vi "系统设置.vi"() -> ()   [LabVIEW 2016]
uses:
  <vilib>/Utility/miscctls.llb/LVPointTypeDef.ctl
  <vilib>/ptbypt/NI_PtbyPt.lvlib
  <vilib>/Utility/config.llb/NI_LVConfig.lvlib
  PLC/PLC.lvlib
panel:
  in  "总磷":bool
  in  "模块启用配置":bool
  in  "短信报警设置":bool
  in  "首页显示设置":bool
  in  "跨度核查":bool
  in  "空白核查":bool
  out "选项卡控件":enum32{"自由设定", "国标协议", "流量设定"}(tab)
  in  "24H周期设置":bool[](xcontrol)
  in  "运行间隔":i16=4 min=1 max=24
  in  "流量阈值":dbl=4.0 min=1.0 max=24.0
  in  "时间阈值":u16=4 min=1 max=24
  in  "周期设置":enum16{"自由设定", "国标协议", "流量设定"}(ring)
  out "x = y?":bool
  in  "质控启动日期":string(combo)="关闭"
  in  "跨度核查时间":u16(ring)=6 items=["00H", "01H", "02H", "03H", "04H", "05H", "06H", "07H", "08H", "09H", "10H", "11H", "12H", "13H", "14H", "15H", "16H", "17H", "18H", "19H", "20H", "21H", "22H", "23H", "关闭"]
  in  "空白核查时间":u16(ring)=2 items=["00H", "01H", "02H", "03H", "04H", "05H", "06H", "07H", "08H", "09H", "10H", "11H", "12H", "13H", "14H", "15H", "16H", "17H", "18H", "19H", "20H", "21H", "22H", "23H", "关闭"]
  in  "CODCr":bool
  in  "总氮":bool
  in  "氨氮":bool
  in  "CODmn":bool
  in  "多参数":bool
  in  "输入密码":dbl
  in  "布尔":bool
  in  "副屏显示设置":bool
  in  "开机启动":bool caption="氨氮禁用"
  in  "运行模式":enum16{"维护模式", "常规模式", "应急模式", "质控模式"}(ring)
  # "注：周期设置分为自由设定和国标协议两种。\n1：选择自由设定情况下：运行间隔将不可选用并变灰色，周期设置可自由手动勾选\n2：选择国标协议情况下：周期时间将由运行间隔选择的时间决定，下方周期设置被禁用并无法手动勾选。\n3：选择流量设定情况下：瞬时流量连续超过流量阈值到达时间阈值设定值，仪器将自动开启测量。"
  # "自动运行启动参数"
  # "质控频次："
  # "零点核查时间："
  # "跨度核查时间："
  # "启动周期设置"
  # "m3/S"
  # "秒"
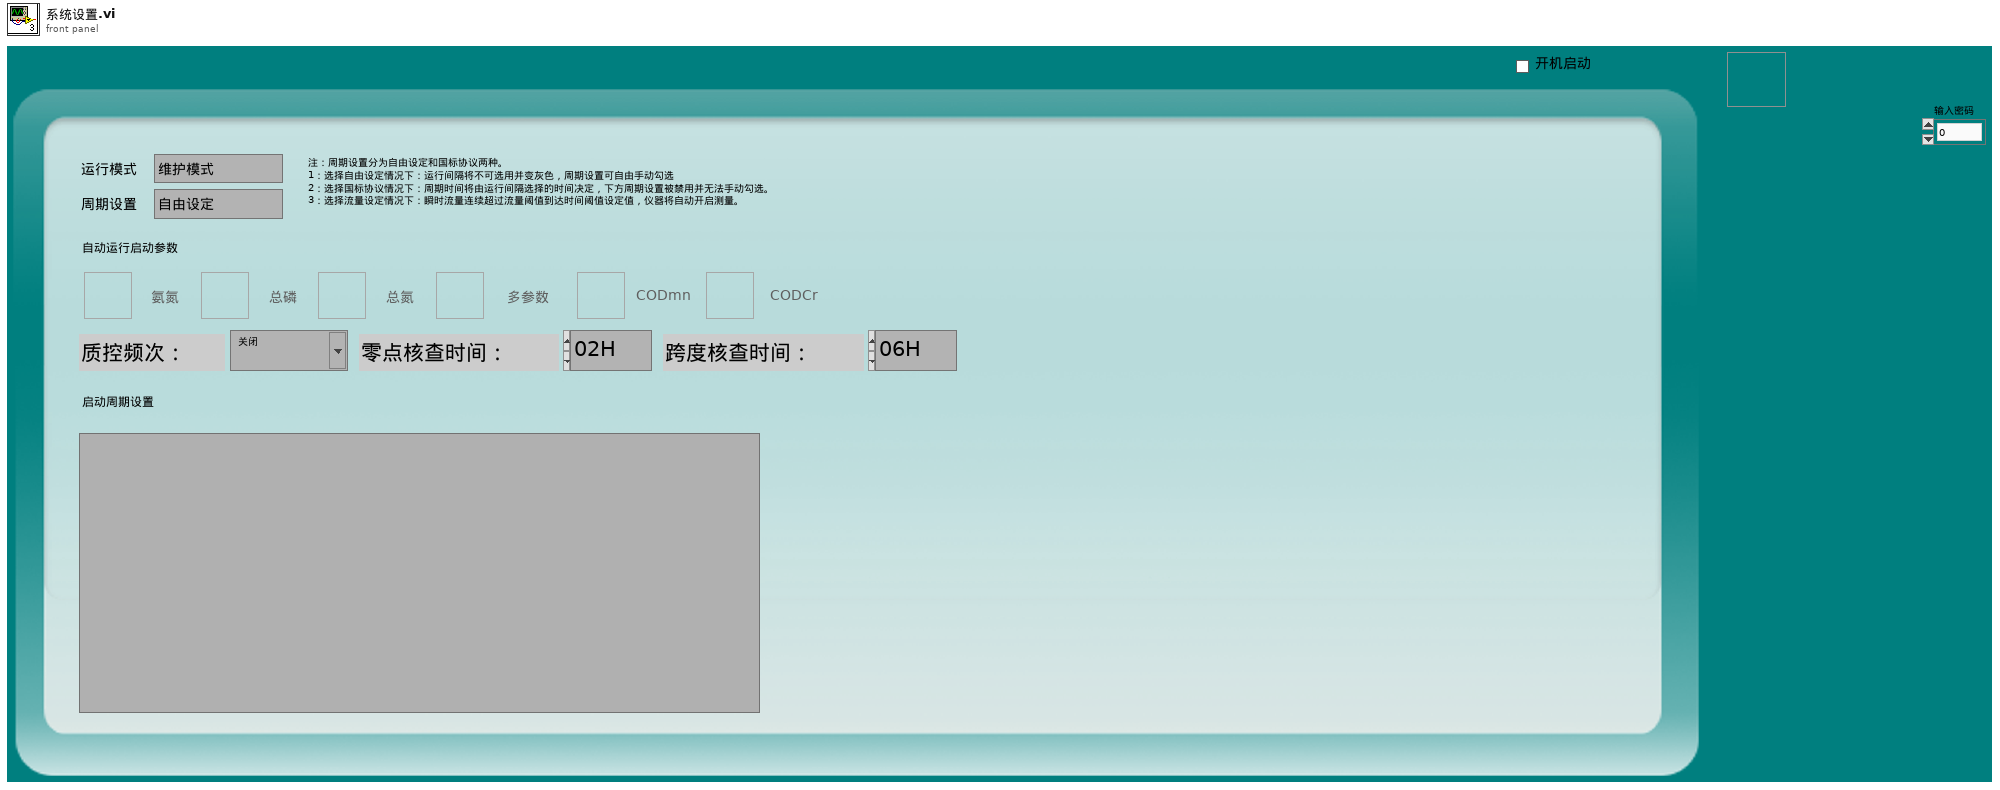
[diagram p1: front panel]
types:
  T1 = typedef "NI_LVConfig.lvlib/Config Data RefNum.ctl" = refnum<k1>
  T2 = typedef "LVPointTypeDef.ctl" = cluster{"Horizontal":i16, "Vertical":i16}
  T3 = enum8{"Enabled", "Disabled", "Disabled and Grayed Out"}
  T4 = enum32{"Bad", "Idle", "Run top level", "Running"}
  T5 = enum32{"Invalid", "Standard", "Closed", "Hidden", "Minimized", "Maximized"}
  T6 = cluster{"运行模式":enum16{"维护模式", "常规模式", "应急模式", "质控模式"}}
  T7 = enum16{"启动测量", "标样核查", "零点核查", "跨度核查", "空白测试", "平行样测试", "加标回收", "空白校准", "标样校准", "初始化（清洗）", "停止测试", "仪器重启", "校时", "模式设置", "测量间隔设置"}
  T8 = cluster{"测量模式":enum16{"水样测量", "标样核查", "零点核查", "跨度核查", "空白测试", "加标回收", "平行样", "校零", "校标"}}
  T9 = cluster{"测试模式":enum16{"正常测试", "集成干预"}, "参数启用":cluster{"氨氮":bool, "总磷":bool, "总氮":bool, "多参数":bool, "CODMn":bool, "CODcr":bool}}
  T10 = cluster{"运行模式":enum16{"维护模式", "常规模式", "应急模式", "质控模式"}, "质控频次":enum16{"关闭", "每天", "星期一", "星期二", "星期三", "星期四", "星期五", "星期六", "星期日"}, "空白核查时间":u16, "跨度核查时间":u16, "24H周期设置":bool[]}
  T11 = typedef "LVDateTimeRec.ctl" = cluster{"秒数的小数部分":dbl, "秒":i32, "分":i32, "时":i32, "日":i32, "月":i32, "年":i32, "天数（周）":i32, "天数（年）":i32, "DST":i32}
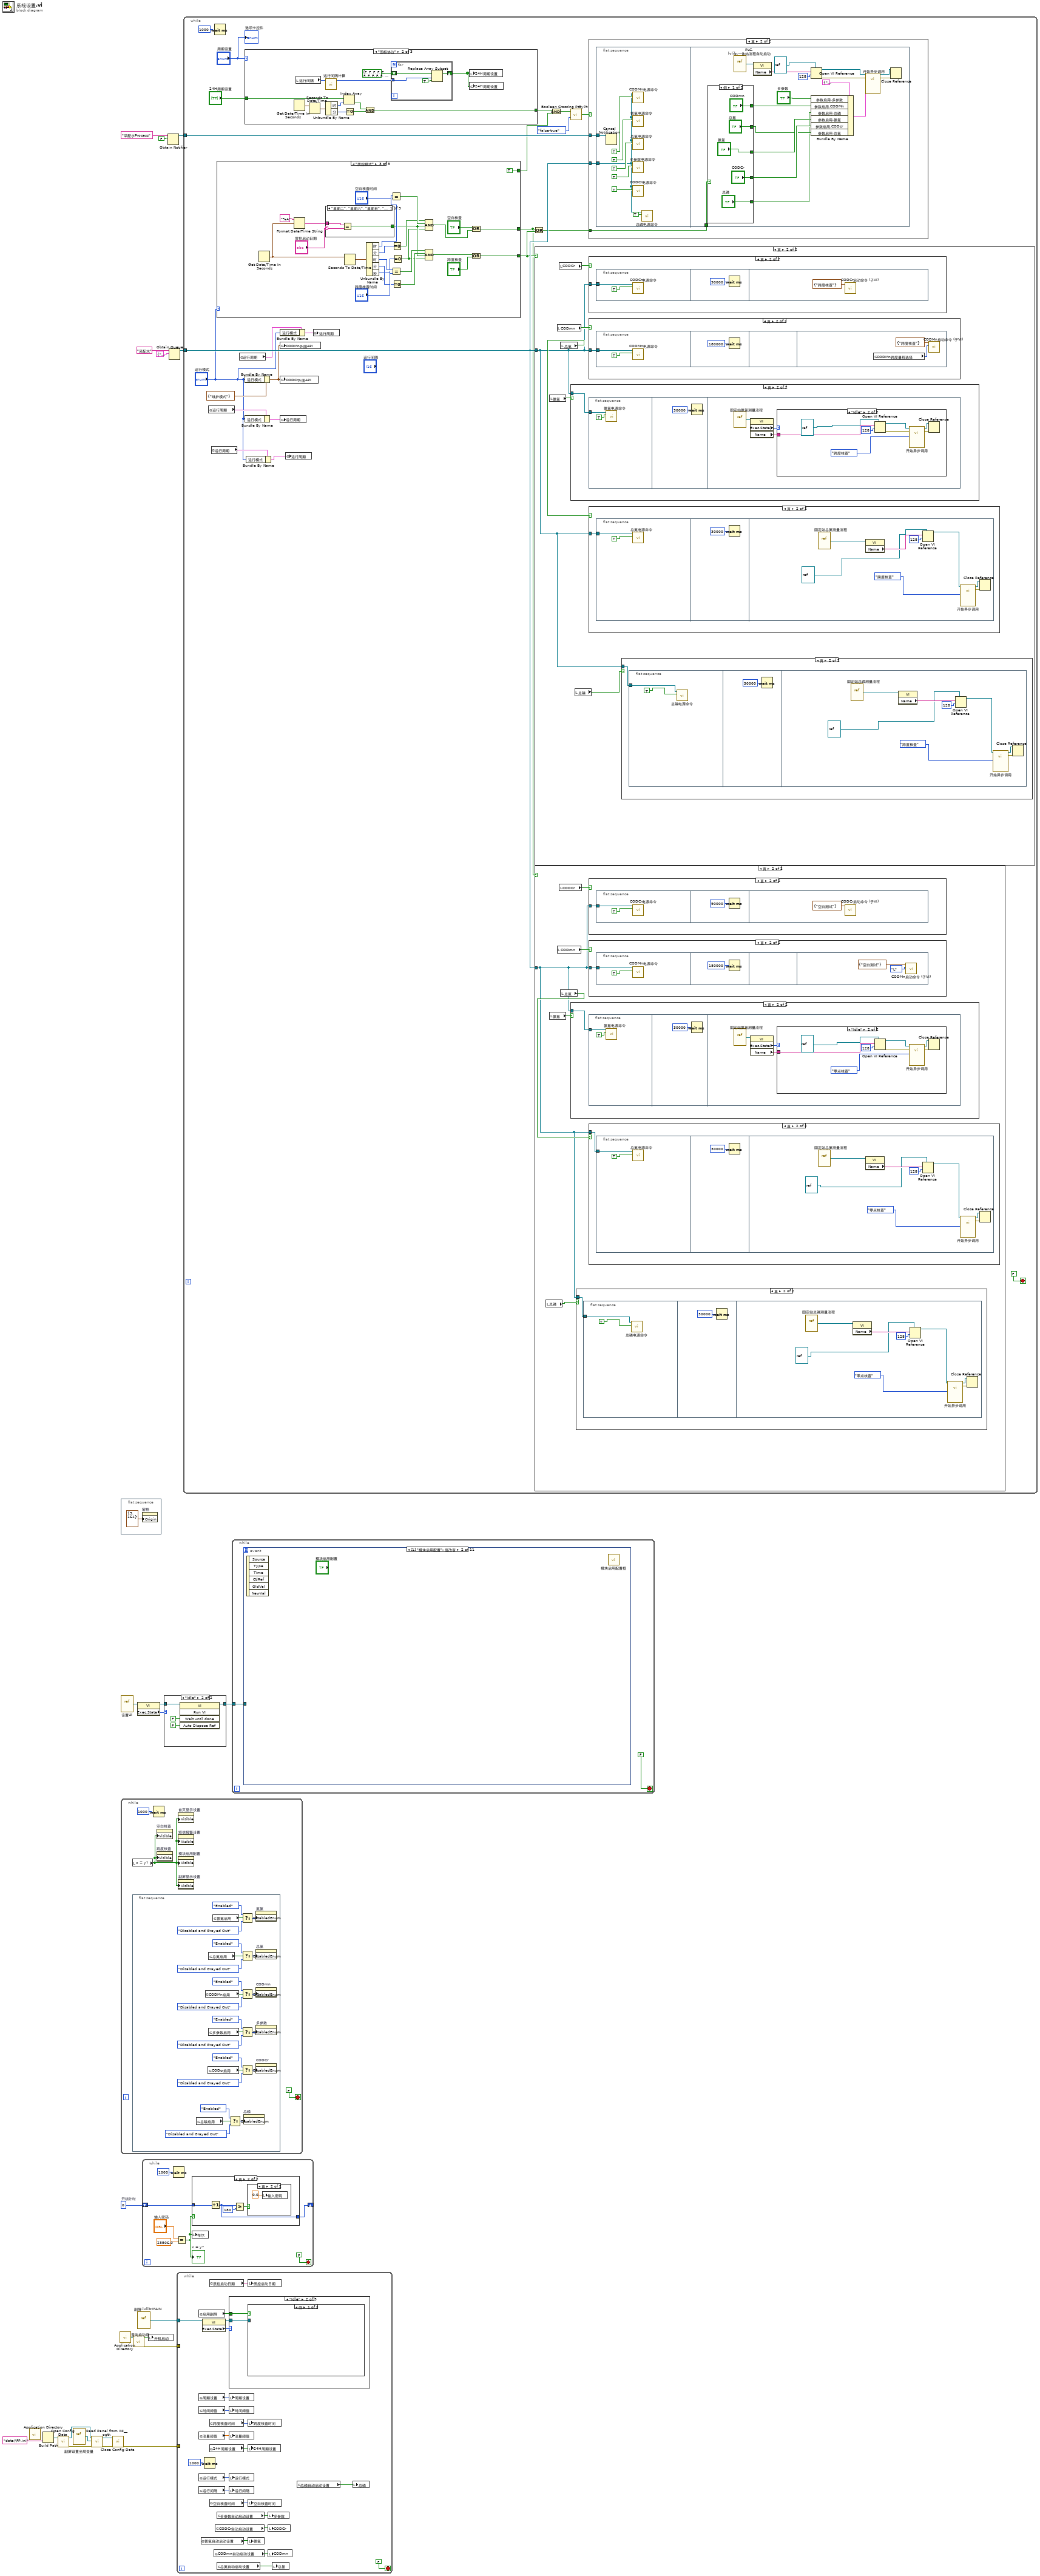
[diagram p0: block diagram]
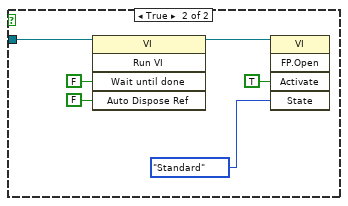
[diagram p6: hidden frame]
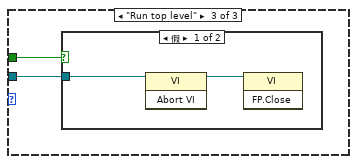
[diagram p7: hidden frame]
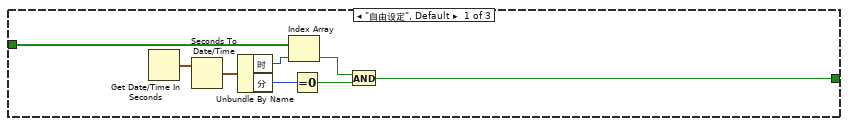
[diagram p9: hidden frame]
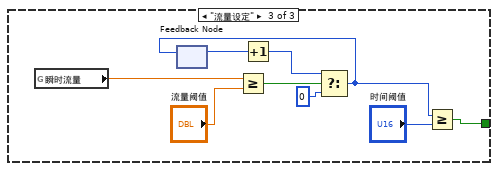
[diagram p10: hidden frame]
diagram:
  w18 = u32 0  # 开锁计时
  n1 = call <vilib>:"Application Directory.vi"() -> ()  [unwired: 1 out]
  n2 = Build Path(name or relative path="data\\FP.ini" ("名称或相对路径")) -> (appended path=w7:path)  [unwired: 1 in]
  n3 = call <vilib>:"Open Config Data.vi"("configuration file path"=w7) -> ("error out"=w6:errorcluster, "refnum"=w3:T1)  [unwired: 8 in, 1 out]
  n4 = vi-ref "副屏设置全局变量.vi"() -> (w4:refnum<vi>)
  n5 = call <userlib>:"Read Panel from INI__ogtk.vi"("error in (no error)"=w6, "VI ref"=w4, "refnum"=w3) -> ("error out"=w5:errorcluster, "refnum out"=w2:T1)  [unwired: 7 in]
  n6 = call <vilib>:"Close Config Data.vi"("error in (no error)"=w5, "refnum"=w2) -> ("error out"=w1:errorcluster)  [unwired: 8 in, 1 out]
  n7 = call <vilib>:"Application Directory.vi"() -> ("Application Directory"=w20:path)
  n8 = flat-sequence {
    frame #0 {
      n9 = property on="窗格" class="Pane"("Origin"=T2 {"Horizontal"=3, "Vertical"=164} ("原点")) -> ()  [unwired: 2 in, 2 out]
    }
  }
  n10 = vi-ref "设置UI.vi"() -> (w13:refnum<vi>)
  n11 = while {
    stop <- FALSE stop-if-true
    n12 = local read "x = y?"() -> (w25:bool)
    n13 = flat-sequence {
      frame #0 {
        n14 = global read "系统设置全局变量.vi" "总磷启用"() -> (w30:bool)
        n15 = global read "系统设置全局变量.vi" "CODMn启用"() -> (w37:bool)
        n16 = global read "系统设置全局变量.vi" "CODcr启用"() -> (w38:bool)
        n17 = global read "系统设置全局变量.vi" "总氮启用"() -> (w39:bool)
        n18 = global read "系统设置全局变量.vi" "多参数启用"() -> (w36:bool)
        n19 = global read "系统设置全局变量.vi" "氨氮启用"() -> (w32:bool)
        n20 = Select(t=T3."Enabled" ("禁用"), s=w30, f=T3."Disabled and Grayed Out" ("禁用")) -> (s? t:f=w31:T3)
        n21 = Select(t=T3."Enabled" ("禁用"), s=w32, f=T3."Disabled and Grayed Out" ("禁用")) -> (s? t:f=w40:T3)
        n22 = Select(t=T3."Enabled" ("禁用"), s=w39, f=T3."Disabled and Grayed Out" ("禁用")) -> (s? t:f=w34:T3)
        n23 = Select(t=T3."Enabled" ("禁用"), s=w37, f=T3."Disabled and Grayed Out" ("禁用")) -> (s? t:f=w41:T3)
        n24 = Select(t=T3."Enabled" ("禁用"), s=w36, f=T3."Disabled and Grayed Out" ("禁用")) -> (s? t:f=w35:T3)
        n25 = Select(t=T3."Enabled" ("禁用"), s=w38, f=T3."Disabled and Grayed Out" ("禁用")) -> (s? t:f=w51:T3)
        n26 = property on="总磷" class="Bool (严格)"("DisabledEnum"=w31) -> ()  [unwired: 2 in, 2 out]
        n27 = property on="氨氮" class="Bool (严格)"("DisabledEnum"=w40) -> ()  [unwired: 2 in, 2 out]
        n28 = property on="总氮" class="Bool (严格)"("DisabledEnum"=w34) -> ()  [unwired: 2 in, 2 out]
        n29 = property on="CODmn" class="Bool (严格)"("DisabledEnum"=w41) -> ()  [unwired: 2 in, 2 out]
        n30 = property on="多参数" class="Bool (严格)"("DisabledEnum"=w35) -> ()  [unwired: 2 in, 2 out]
        n31 = property on="CODCr" class="Bool (严格)"("DisabledEnum"=w51) -> ()  [unwired: 2 in, 2 out]
      }
    }
    n32 = Wait (ms)(milliseconds to wait=u32 1000 ("等待时间（毫秒）")) -> ()  [unwired: 1 out]
    n33 = property on="空白核查" class="Bool"("Visible"=w25) -> ()  [unwired: 2 in, 2 out]
    n34 = property on="跨度核查" class="Bool"("Visible"=w25) -> ()  [unwired: 2 in, 2 out]
    n35 = property on="首页显示设置" class="Bool"("Visible"=w25) -> ()  [unwired: 2 in, 2 out]
    n36 = property on="短信报警设置" class="Bool"("Visible"=w25) -> ()  [unwired: 2 in, 2 out]
    n37 = property on="模块启用配置" class="Bool"("Visible"=w25) -> ()  [unwired: 2 in, 2 out]
    n38 = property on="副屏显示设置" class="Bool"("Visible"=w25) -> ()  [unwired: 2 in, 2 out]
  }
  n39 = call "查询启动项.vi"("启动文件路径"=w20) -> ("error out"=w9:errorcluster, "包含启动项"=w19:bool)  [unwired: 9 in]
  n40 = property class="VI"(reference=w13) -> (reference out=w11:refnum<vi>, "Exec.State"=w12:T4)  [unwired: 1 in, 1 out]
  n41 = vi-ref "副屏.lvlib:MAIN.vi"() -> (w14:refnum<vi>)
  n42 = while {
    shift-right: [w53] -> _
    shift-left: w18 -> [w54]
    stop <- FALSE stop-if-true
    n43 = Wait (ms)(milliseconds to wait=u32 1000 ("等待时间（毫秒）")) -> ()  [unwired: 1 out]
    n44 = Equal?(x="输入密码", y=23506.0) -> (x = y?=w52:bool)
    "x = y?" <- w52
    n45 = case shown="真" w52 {
      tunnel: w54 -> [_ w62]
      tunnel: [_ w61] -> w53
      frame False {
      }
      frame True {
        n46 = Increment(x=w62) -> (x+1=w61:u32)
        n47 = Greater Or Equal?(x=w61, y=u32 180) -> (x >= y?=w59:bool)
        n48 = case shown="真" w59 {
          frame False {
          }
          frame True {
            n49 = local write "输入密码"(0.0 ("输入密码")) -> ()
          }
        }
      }
    }
    n50 = local write "布尔"(w52) -> ()
  }
  n51 = local write "开机启动"(w19) -> ()
  n52 = case shown="\"Idle\"" w12 {
    tunnel: w11 -> [w64 w68]
    tunnel: [w64 w67] -> w10
    frame "Bad", Default {
    }
    frame "Idle" {
      n53 = invoke class="VI" method="Run VI"(reference=w68, "Wait until done"=FALSE ("结束前等待"), "Auto Dispose Ref"=FALSE ("自动销毁引用")) -> (reference out=w67:refnum<vi>)  [unwired: 2 in, 4 out]
    }
  }
  n54 = Obtain Notifier(name (unnamed)="采配水Process" ("名称（未命名）"), notification data type=FALSE) -> (notifier out=w21:refnum<notifier>)  [unwired: 2 in, 2 out]
  n55 = Obtain Queue(name (unnamed)="采配水" ("名称（未命名）"), element data type=cluster{"命令":string, "数据":variant} {"命令"="", "数据"=variant}) -> (queue out=w15:refnum<queue>)  [unwired: 3 in, 2 out]
  n56 = while {
    tunnel: w14 -> [w81]
    tunnel: w9 -> [_]
    tunnel: w1 -> [_]
    stop <- FALSE stop-if-true
    n57 = global read "副屏设置全局变量.vi" "启用副屏"() -> (w79:bool)
    n58 = global read "系统设置全局变量.vi" "周期设置"() -> (w74:enum16{"自由设定", "国标协议", "流量设定"})
    n59 = global read "系统设置全局变量.vi" "时间阈值"() -> (w70:u16)
    n60 = global read "系统设置全局变量.vi" "流量阈值"() -> (w71:dbl)
    n61 = global read "系统设置全局变量.vi" "运行模式"() -> (w72:enum16{"维护模式", "常规模式", "应急模式", "质控模式"})
    n62 = global read "系统设置全局变量.vi" "运行间隔"() -> (w73:i16)
    n63 = global read "系统设置全局变量.vi" "氨氮自动启动设置"() -> (w86:bool)
    n64 = property class="VI"(reference=w81) -> (reference out=w78:refnum<vi>, "Exec.State"=w80:T4)  [unwired: 1 in, 1 out]
    n65 = Wait (ms)(milliseconds to wait=u32 1000 ("等待时间（毫秒）")) -> ()  [unwired: 1 out]
    n66 = global read "系统设置全局变量.vi" "质控启动日期"() -> (w77:string)
    n67 = global read "系统设置全局变量.vi" "跨度核查时间"() -> (w75:u16)
    n68 = global read "系统设置全局变量.vi" "24H周期设置"() -> (w87:bool[])
    n69 = global read "系统设置全局变量.vi" "空白核查时间"() -> (w76:u16)
    n70 = global read "系统设置全局变量.vi" "CODmn自动启动设置"() -> (w83:bool)
    n71 = global read "系统设置全局变量.vi" "CODCr自动启动设置"() -> (w85:bool)
    n72 = global read "系统设置全局变量.vi" "多参数自动启动设置"() -> (w82:bool)
    n73 = global read "系统设置全局变量.vi" "总氮自动启动设置"() -> (w84:bool)
    n74 = case shown="\"Idle\"" w80 {
      tunnel: w79 -> [_ w90 w98]
      tunnel: w78 -> [_ w91 w99]
      frame "Bad", Default {
      }
      frame "Idle" {
        n75 = case shown="假" w90 {
          tunnel: w91 -> [_ w97]
          frame False {
          }
          frame True {
            n76 = invoke class="VI" method="Run VI"(reference=w97, "Wait until done"=FALSE ("结束前等待"), "Auto Dispose Ref"=FALSE ("自动销毁引用")) -> (reference out=w92:refnum<vi>)  [unwired: 2 in, 4 out]
            n77 = invoke class="VI" method="FP.Open"(reference=w92, "Activate"=TRUE ("激活？"), "State"=T5."Standard" ("状态")) -> ()  [unwired: 2 in, 5 out]
          }
        }
      }
      frame "Run top level" {
        n78 = case shown="假" w98 {
          tunnel: w99 -> [w100 _]
          frame False {
            n79 = invoke class="VI" method="Abort VI"(reference=w100) -> (reference out=w101:refnum<vi>)  [unwired: 2 in, 2 out]
            n80 = invoke class="VI" method="FP.Close"(reference=w101) -> ()  [unwired: 2 in, 3 out]
          }
          frame True {
          }
        }
      }
    }
    n81 = local write "周期设置"(w74) -> ()
    n82 = local write "时间阈值"(w70) -> ()
    n83 = local write "流量阈值"(w71) -> ()
    n84 = local write "运行模式"(w72) -> ()
    n85 = local write "运行间隔"(w73) -> ()
    n86 = local write "质控启动日期"(w77) -> ()
    n87 = local write "跨度核查时间"(w75) -> ()
    n88 = local write "24H周期设置"(w87) -> ()
    n89 = local write "空白核查时间"(w76) -> ()
    n90 = local write "氨氮"(w86) -> ()
    n91 = local write "多参数"(w82) -> ()
    n92 = local write "CODCr"(w85) -> ()
    n93 = local write "CODmn"(w83) -> ()
    n94 = local write "总氮"(w84) -> ()
    n95 = global read "系统设置全局变量.vi" "总磷自动启动设置"() -> (w69:bool)
    n96 = local write "总磷"(w69) -> ()
  }
  n97 = while {
    tunnel: w21 -> [w122]
    tunnel: w15 -> [w118]
    stop <- FALSE stop-if-true
    n98 = global read "总氮断电保存全局变量.vi" "运行周期"() -> (w106:T10)
    n99 = global read "总磷断电保存全局变量.vi" "运行周期"() -> (w104:T10)
    n100 = Wait (ms)(milliseconds to wait=u32 1000 ("等待时间（毫秒）")) -> ()  [unwired: 1 out]
    n101 = case shown="\"质控模式\"" "运行模式" {
      tunnel: [_ _ w304] -> w111
      tunnel: [_ _ w308] -> w110
      tunnel: [_ TRUE TRUE] -> w115
      frame "维护模式", Default {
      }
      frame "常规模式" {
      }
      frame "质控模式" {
        n102 = Get Date/Time In Seconds() -> (seconds since 1Jan1904=w315:timestamp)
        n103 = Format Date/Time String(time format string (%c)="%A" ("时间格式字符串(%c)"), seconds (now)=w315) -> (date/time string=w313:string)  [unwired: 1 in]
        n104 = case shown="\"星期二\", \"星期六\", \"星期日\", \"星期三\", \"星期四\", \"星期五\", \"星期一\"" "质控启动日期" {
          selector: "质控启动日期" -> [w331 _ _]
          tunnel: [w330 TRUE FALSE] -> w316
          tunnel: w313 -> [w329 _ _]
          frame "星期二", "星期六", "星期日", "星期三", "星期四", "星期五", "星期一" {
            n105 = Equal?(x=w329, y=w331) -> (x = y?=w330:bool)
          }
          frame "每天" {
          }
          frame "关闭", Default {
          }
        }
        n106 = Seconds To Date/Time(time stamp (now)=w315) -> (date time rec=w328:T11)  [unwired: 1 in]
        n107 = Unbundle By Name(w328) -> ("时"=w327:i32, "分"=w325:i32, "时"=w321:i32, "分"=w320:i32, "秒"=w312:i32)
        n108 = Equal?(x=w327, y="空白核查时间") -> (x = y?=w324:bool)
        n109 = Equal?(x=w321, y="跨度核查时间") -> (x = y?=w319:bool)
        n110 = Equal To 0?(x=w325) -> (x = 0?=w323:bool)
        n111 = Equal To 0?(x=w320) -> (x = 0?=w318:bool)
        n112 = Equal To 0?(x=w312) -> (x = 0?=w311:bool)
        n113 = Compound Arithmetic op=AND ("复合运算")(w323, w324, w316, w311) -> (w309:bool)
        n114 = Compound Arithmetic op=AND ("复合运算")(w319, w318, w316, w311) -> (w306:bool)
        n115 = Or(x="空白核查", y=w309) -> (x .or. y?=w308:bool)
        n116 = Or(x=w306, y="跨度核查") -> (x .or. y?=w304:bool)
      }
    }
    n117 = global read "氨氮断电保存全局变量.vi" "运行周期"() -> (w108:T10)
    n118 = case shown="\"国标协议\"" "周期设置" {
      tunnel: [w126 w133 w149] -> w114
      tunnel: "24H周期设置" -> [w125 w134 _]
      frame "自由设定", Default {
        n119 = Get Date/Time In Seconds() -> (seconds since 1Jan1904=w127:timestamp)
        n120 = Seconds To Date/Time(time stamp (now)=w127) -> (date time rec=w128:T11)  [unwired: 1 in]
        n121 = Unbundle By Name(w128) -> ("时"=w131:i32, "分"=w129:i32)
        n122 = Index Array(array=w125, index=w131) -> (element=w132:bool)
        n123 = Equal To 0?(x=w129) -> (x = 0?=w130:bool)
        n124 = And(x=w132, y=w130) -> (x .and. y?=w126:bool)
      }
      frame "国标协议" {
        n125 = Get Date/Time In Seconds() -> (seconds since 1Jan1904=w135:timestamp)
        n126 = local read "运行间隔"() -> (w144:i16)
        n127 = Seconds To Date/Time(time stamp (now)=w135) -> (date time rec=w136:T11)  [unwired: 1 in]
        n128 = call "运行间隔计算.vi"("运行周期"=w144) -> ("数组"=w143:i32[])  [unwired: 10 in]
        n129 = Unbundle By Name(w136) -> ("时"=w139:i32, "分"=w137:i32)
        n130 = Index Array(array=w134, index=w139) -> (element=w140:bool)
        n131 = Equal To 0?(x=w137) -> (x = 0?=w138:bool)
        n132 = And(x=w140, y=w138) -> (x .and. y?=w133:bool)
        n133 = for {
          tunnel: w143 -> [w147] mode=indexing
          shift-right: [w145] -> w141
          shift-left: bool[] [FALSE, FALSE, FALSE, FALSE, FALSE, FALSE, FALSE, FALSE, FALSE, FALSE, FALSE, FALSE, FALSE, FALSE, FALSE, FALSE, FALSE, FALSE, FALSE, FALSE, FALSE, FALSE, FALSE, FALSE] ("24H周期设置") -> [w148]
          n134 = Replace Array Subset(array=w148, new element=TRUE ("新元素/子数组"), index=w147) -> (w145:bool[])
        }
        n135 = local write "24H周期设置"(w141) -> ()
        n136 = global write "系统设置全局变量.vi" "24H周期设置"(w141) -> ()
      }
      frame "流量设定" {
        n137 = global read "流量计全局变量.vi" "瞬时流量"() -> (w157:dbl)
        n138 = feedback #1() -> (w154:i16)  [unwired: 1 in]
        n139 = Greater Or Equal?(x=w157, y="流量阈值") -> (x >= y?=w152:bool)
        n140 = Increment(x=w154) -> (x+1=w153:i16)
        n141 = Select(t=w153, s=w152, f=i16 0) -> (s? t:f=w151:i16)
        n142 = feedback-in #1(w151) -> ()
        n143 = Greater Or Equal?(x=w151, y="时间阈值") -> (x >= y?=w149:bool)
      }
    }
    n144 = Bundle By Name(cluster=T6 {"运行模式"=enum."维护模式"} ("外围API"), "运行模式"="运行模式") -> (w112:T6)
    n145 = Bundle By Name(cluster=w106, "运行模式"="运行模式") -> (w105:T10)
    n146 = Bundle By Name(cluster=w104, "运行模式"="运行模式") -> (w103:T10)
    n147 = Bundle By Name(cluster=w108, "运行模式"="运行模式") -> (w107:T10)
    n148 = global write "CODMN外部API.vi" "CODMn外围API"(w112) -> ()
    n149 = global write "CODCr外部API.vi" "CODCr外围API"(w112) -> ()
    n150 = global write "总氮断电保存全局变量.vi" "运行周期"(w105) -> ()
    n151 = global write "总磷断电保存全局变量.vi" "运行周期"(w103) -> ()
    n152 = global write "氨氮断电保存全局变量.vi" "运行周期"(w107) -> ()
    n153 = Or(x=w110, y=w111) -> (x .or. y?=w109:bool)
    n154 = case shown="真" w111 {
      tunnel: w118 -> [_ w159]
      frame False {
      }
      frame True {
        n155 = local read "氨氮"() -> (w163:bool)
        n156 = local read "CODmn"() -> (w161:bool)
        n157 = local read "CODCr"() -> (w160:bool)
        n158 = local read "总氮"() -> (w162:bool)
        n159 = case shown="真" w163 {
          tunnel: w159 -> [_ w199]
          frame False {
          }
          frame True {
            n160 = flat-sequence {
              tunnel: w199 -> [w200]
              frame #0 {
                n161 = call "氨氮电源命令.vi"("通电/断电"=TRUE, "队列"=w200) -> ()  [unwired: 9 in, 1 out]
              }
              frame #1 {
                n162 = Wait (ms)(milliseconds to wait=u32 30000 ("等待时间（毫秒）")) -> ()  [unwired: 1 out]
              }
              frame #2 {
                n163 = vi-ref "固定站氨氮测量流程.vi"() -> (w205:refnum<vi>)
                n164 = property class="VI"(reference=w205) -> ("Exec.State"=w203:T4, "Name"=w204:string)  [unwired: 1 in, 2 out]
                n165 = case shown="\"Idle\"" w203 {
                  tunnel: w204 -> [_ w210]
                  frame "Bad", Default {
                  }
                  frame "Idle" {
                    n166 = Open VI Reference(type specifier VI Refnum (for type only)=refnum<vi> refnum, vi path=w210, options=128 ("选项")) -> (vi reference=w208:refnum<vi>, error out=w211:errorcluster)  [unwired: 3 in]
                    n167 = call-by-ref "开始异步调用"(reference=w208, error in=w211, "控制命令"=T7."跨度核查") -> (reference out=w212:refnum<vi>, error out=w213:errorcluster)  [unwired: 11 in]
                    n168 = Close Reference(reference=w212, error in (no error)=w213) -> ()  [unwired: 1 out]
                  }
                }
              }
            }
          }
        }
        n169 = local read "总磷"() -> (w158:bool)
        n170 = case shown="真" w160 {
          tunnel: w159 -> [_ w176]
          frame False {
          }
          frame True {
            n171 = flat-sequence {
              tunnel: w176 -> [w177]
              frame #0 {
                n172 = call "CODCr电源命令.vi"("通电/断电"=TRUE, "队列"=w177) -> ()  [unwired: 9 in, 1 out]
              }
              frame #1 {
                n173 = Wait (ms)(milliseconds to wait=u32 90000 ("等待时间（毫秒）")) -> ()  [unwired: 1 out]
              }
              frame #2 {
                n174 = call "CODCr启动命令 (子VI).vi"("启动测量模式"=T8 {"测量模式"=enum."跨度核查"}) -> ()  [unwired: 11 in]
              }
            }
          }
        }
        n175 = case shown="真" w161 {
          tunnel: w159 -> [_ w181]
          frame False {
          }
          frame True {
            n176 = flat-sequence {
              tunnel: w181 -> [w182]
              frame #0 {
                n177 = call "CODMn电源命令.vi"("通电/断电"=TRUE, "队列"=w182) -> ()  [unwired: 9 in, 1 out]
              }
              frame #1 {
                n178 = Wait (ms)(milliseconds to wait=u32 180000 ("等待时间（毫秒）")) -> ()  [unwired: 1 out]
              }
              frame #2 {
              }
              frame #3 {
                n179 = global read "CODMn断电保存全局变量.vi" "CODMn跨度量程选择"() -> (w185:enum32{"H", "L", "AUTO"})
                n180 = call "CODMn启动命令 (子VI).vi"("CODMn量程切换"=w185, "启动测量模式"=T8 {"测量模式"=enum."跨度核查"}) -> ()  [unwired: 10 in]
              }
            }
          }
        }
        n181 = case shown="真" w162 {
          tunnel: w159 -> [_ w187]
          frame False {
          }
          frame True {
            n182 = flat-sequence {
              tunnel: w187 -> [w189]
              frame #0 {
                n183 = call "总氮电源命令.vi"("通电/断电"=TRUE, "队列"=w189) -> ()  [unwired: 9 in, 1 out]
              }
              frame #1 {
                n184 = Wait (ms)(milliseconds to wait=u32 30000 ("等待时间（毫秒）")) -> ()  [unwired: 1 out]
              }
              frame #2 {
                n185 = vi-ref "固定站总氮测量流程.vi"() -> (w196:refnum<vi>)
                n186 = property class="VI"(reference=w196) -> ("Name"=w197:string)  [unwired: 1 in, 2 out]
                n187 = Open VI Reference(type specifier VI Refnum (for type only)=refnum<vi> refnum, vi path=w197, options=128 ("选项")) -> (vi reference=w195:refnum<vi>)  [unwired: 3 in, 1 out]
                n188 = call-by-ref "开始异步调用"(reference=w195, "控制命令"=T7."跨度核查") -> (reference out=w194:refnum<vi>, error out=w193:errorcluster)  [unwired: 12 in]
                n189 = Close Reference(reference=w194, error in (no error)=w193) -> ()  [unwired: 1 out]
              }
            }
          }
        }
        n190 = case shown="真" w158 {
          tunnel: w159 -> [_ w164]
          frame False {
          }
          frame True {
            n191 = flat-sequence {
              tunnel: w164 -> [w166]
              frame #0 {
                n192 = call "总磷电源命令.vi"("通电/断电"=TRUE, "队列"=w166) -> ()  [unwired: 9 in, 1 out]
              }
              frame #1 {
                n193 = Wait (ms)(milliseconds to wait=u32 30000 ("等待时间（毫秒）")) -> ()  [unwired: 1 out]
              }
              frame #2 {
                n194 = vi-ref "固定站总磷测量流程.vi"() -> (w173:refnum<vi>)
                n195 = property class="VI"(reference=w173) -> ("Name"=w174:string)  [unwired: 1 in, 2 out]
                n196 = Open VI Reference(type specifier VI Refnum (for type only)=refnum<vi> refnum, vi path=w174, options=128 ("选项")) -> (vi reference=w172:refnum<vi>)  [unwired: 3 in, 1 out]
                n197 = call-by-ref "开始异步调用"(reference=w172, "控制命令"=T7."跨度核查") -> (reference out=w171:refnum<vi>, error out=w170:errorcluster)  [unwired: 12 in]
                n198 = Close Reference(reference=w171, error in (no error)=w170) -> ()  [unwired: 1 out]
              }
            }
          }
        }
      }
    }
    n199 = case shown="真" w110 {
      tunnel: w118 -> [_ w215]
      frame False {
      }
      frame True {
        n200 = local read "总磷"() -> (w214:bool)
        n201 = local read "氨氮"() -> (w219:bool)
        n202 = local read "CODmn"() -> (w217:bool)
        n203 = local read "CODCr"() -> (w216:bool)
        n204 = local read "总氮"() -> (w218:bool)
        n205 = case shown="真" w219 {
          tunnel: w215 -> [_ w255]
          frame False {
          }
          frame True {
            n206 = flat-sequence {
              tunnel: w255 -> [w256]
              frame #0 {
                n207 = call "氨氮电源命令.vi"("通电/断电"=TRUE, "队列"=w256) -> ()  [unwired: 9 in, 1 out]
              }
              frame #1 {
                n208 = Wait (ms)(milliseconds to wait=u32 30000 ("等待时间（毫秒）")) -> ()  [unwired: 1 out]
              }
              frame #2 {
                n209 = vi-ref "固定站氨氮测量流程.vi"() -> (w261:refnum<vi>)
                n210 = property class="VI"(reference=w261) -> ("Exec.State"=w259:T4, "Name"=w260:string)  [unwired: 1 in, 2 out]
                n211 = case shown="\"Idle\"" w259 {
                  tunnel: w260 -> [_ w266]
                  frame "Bad", Default {
                  }
                  frame "Idle" {
                    n212 = Open VI Reference(type specifier VI Refnum (for type only)=refnum<vi> refnum, vi path=w266, options=128 ("选项")) -> (vi reference=w264:refnum<vi>, error out=w267:errorcluster)  [unwired: 3 in]
                    n213 = call-by-ref "开始异步调用"(reference=w264, error in=w267, "控制命令"=T7."零点核查") -> (reference out=w268:refnum<vi>, error out=w269:errorcluster)  [unwired: 11 in]
                    n214 = Close Reference(reference=w268, error in (no error)=w269) -> ()  [unwired: 1 out]
                  }
                }
              }
            }
          }
        }
        n215 = case shown="真" w214 {
          tunnel: w215 -> [_ w220]
          frame False {
          }
          frame True {
            n216 = flat-sequence {
              tunnel: w220 -> [w222]
              frame #0 {
                n217 = call "总磷电源命令.vi"("通电/断电"=TRUE, "队列"=w222) -> ()  [unwired: 9 in, 1 out]
              }
              frame #1 {
                n218 = Wait (ms)(milliseconds to wait=u32 30000 ("等待时间（毫秒）")) -> ()  [unwired: 1 out]
              }
              frame #2 {
                n219 = vi-ref "固定站总磷测量流程.vi"() -> (w229:refnum<vi>)
                n220 = property class="VI"(reference=w229) -> ("Name"=w230:string)  [unwired: 1 in, 2 out]
                n221 = Open VI Reference(type specifier VI Refnum (for type only)=refnum<vi> refnum, vi path=w230, options=128 ("选项")) -> (vi reference=w228:refnum<vi>)  [unwired: 3 in, 1 out]
                n222 = call-by-ref "开始异步调用"(reference=w228, "控制命令"=T7."零点核查") -> (reference out=w227:refnum<vi>, error out=w226:errorcluster)  [unwired: 12 in]
                n223 = Close Reference(reference=w227, error in (no error)=w226) -> ()  [unwired: 1 out]
              }
            }
          }
        }
        n224 = case shown="真" w216 {
          tunnel: w215 -> [_ w232]
          frame False {
          }
          frame True {
            n225 = flat-sequence {
              tunnel: w232 -> [w233]
              frame #0 {
                n226 = call "CODCr电源命令.vi"("通电/断电"=TRUE, "队列"=w233) -> ()  [unwired: 9 in, 1 out]
              }
              frame #1 {
                n227 = Wait (ms)(milliseconds to wait=u32 90000 ("等待时间（毫秒）")) -> ()  [unwired: 1 out]
              }
              frame #2 {
                n228 = call "CODCr启动命令 (子VI).vi"("启动测量模式"=T8 {"测量模式"=enum."空白测试"}) -> ()  [unwired: 11 in]
              }
            }
          }
        }
        n229 = case shown="真" w217 {
          tunnel: w215 -> [_ w237]
          frame False {
          }
          frame True {
            n230 = flat-sequence {
              tunnel: w237 -> [w238]
              frame #0 {
                n231 = call "CODMn电源命令.vi"("通电/断电"=TRUE, "队列"=w238) -> ()  [unwired: 9 in, 1 out]
              }
              frame #1 {
                n232 = Wait (ms)(milliseconds to wait=u32 180000 ("等待时间（毫秒）")) -> ()  [unwired: 1 out]
              }
              frame #2 {
              }
              frame #3 {
                n233 = call "CODMn启动命令 (子VI).vi"("CODMn量程切换"=enum32{"H", "L", "AUTO"}."L", "启动测量模式"=T8 {"测量模式"=enum."空白测试"}) -> ()  [unwired: 10 in]
              }
            }
          }
        }
        n234 = case shown="真" w218 {
          tunnel: w215 -> [_ w243]
          frame False {
          }
          frame True {
            n235 = flat-sequence {
              tunnel: w243 -> [w245]
              frame #0 {
                n236 = call "总氮电源命令.vi"("通电/断电"=TRUE, "队列"=w245) -> ()  [unwired: 9 in, 1 out]
              }
              frame #1 {
                n237 = Wait (ms)(milliseconds to wait=u32 30000 ("等待时间（毫秒）")) -> ()  [unwired: 1 out]
              }
              frame #2 {
                n238 = vi-ref "固定站总氮测量流程.vi"() -> (w252:refnum<vi>)
                n239 = property class="VI"(reference=w252) -> ("Name"=w253:string)  [unwired: 1 in, 2 out]
                n240 = Open VI Reference(type specifier VI Refnum (for type only)=refnum<vi> refnum, vi path=w253, options=128 ("选项")) -> (vi reference=w251:refnum<vi>)  [unwired: 3 in, 1 out]
                n241 = call-by-ref "开始异步调用"(reference=w251, "控制命令"=T7."零点核查") -> (reference out=w250:refnum<vi>, error out=w249:errorcluster)  [unwired: 12 in]
                n242 = Close Reference(reference=w250, error in (no error)=w249) -> ()  [unwired: 1 out]
              }
            }
          }
        }
      }
    }
    n243 = And(x=w114, y=w115) -> (x .and. y?=w113:bool)
    n244 = call <vilib>:"Boolean Crossing PtByPt.vi"("direction"=enum16{"either", "false-true", "true-false"}."false-true", "input"=w113) -> ("crossing"=w120:bool)  [unwired: 1 in]
    n245 = case shown="真" w120 {
      tunnel: w122 -> [_ w272]
      tunnel: w118 -> [_ w271]
      tunnel: w109 -> [_ w270]
      frame False {
      }
      frame True {
        n246 = flat-sequence {
          tunnel: w272 -> [w280]
          tunnel: w271 -> [w274]
          tunnel: w270 -> [w286]
          frame #0 {
            n247 = Cancel Notification(0:w280) -> ()  [unwired: 1 in, 3 out]
            n248 = call "CODMn电源命令.vi"("通电/断电"=TRUE, "队列"=w274) -> ()  [unwired: 9 in, 1 out]
            n249 = call "氨氮电源命令.vi"("通电/断电"=TRUE, "队列"=w274) -> ()  [unwired: 9 in, 1 out]
            n250 = call "总氮电源命令.vi"("通电/断电"=TRUE, "队列"=w274) -> ()  [unwired: 9 in, 1 out]
            n251 = call "多参数电源命令.vi"("通电/断电"=TRUE, "队列"=w274) -> ()  [unwired: 9 in, 1 out]
            n252 = call "CODCr电源命令.vi"("通电/断电"=TRUE, "队列"=w274) -> ()  [unwired: 9 in, 1 out]
            n253 = call "总磷电源命令.vi"("通电/断电"=TRUE, "队列"=w274) -> ()  [unwired: 9 in, 1 out]
          }
          frame #1 {
            n254 = case shown="假" w286 {
              tunnel: ["CODmn" _] -> w296
              tunnel: ["总氮" _] -> w282
              tunnel: ["CODCr" _] -> w295
              tunnel: ["氨氮" _] -> w294
              tunnel: ["总磷" _] -> w281
              frame False {
              }
              frame True {
              }
            }
            n255 = vi-ref "PLC.lvlib:一体站流程自动启动.vi"() -> (w291:refnum<vi>)
            n256 = property class="VI"(reference=w291) -> ("Name"=w292:string)  [unwired: 1 in, 2 out]
            n257 = Open VI Reference(type specifier VI Refnum (for type only)=refnum<vi> refnum, vi path=w292, options=128 ("选项")) -> (vi reference=w290:refnum<vi>, error out=w289:errorcluster)  [unwired: 3 in]
            n258 = Bundle By Name(cluster=T9 {"测试模式"=enum."正常测试", "参数启用"={"氨氮"=FALSE, "总磷"=FALSE, "总氮"=FALSE, "多参数"=FALSE, "CODMn"=FALSE, "CODcr"=FALSE}} ("参数"), "参数启用.多参数"="多参数", "参数启用.CODMn"=w296, "参数启用.总磷"=w281, "参数启用.氨氮"=w294, "参数启用.CODcr"=w295, "参数启用.总氮"=w282) -> (w283:T9)
            n259 = call-by-ref "开始异步调用"(reference=w290, error in=w289, "参数"=w283) -> (reference out=w288:refnum<vi>, error out=w287:errorcluster)  [unwired: 11 in]
            n260 = Close Reference(reference=w288, error in (no error)=w287) -> ()  [unwired: 1 out]
          }
        }
      }
    }
    "选项卡控件" <- "周期设置"
  }
  n261 = while {
    tunnel: w10 -> [w334]
    stop <- FALSE stop-if-true
    n262 = event shown="[1] \"模块启用配置\": 值改变" {
      selector: _ -> [_ _ _ _ _ _ _ _ _ _ _]
      dyn-events: _ -> [_ _ _ _ _ _ _ _ _ _ _]
      timeout: _ -> [_ _ _ _ _ _ _ _ _ _ _]
      tunnel: w334 -> [_ _ _ _ _ _ _ _ _ w389 _]
      event Timeout {
        n263 = event-data() -> ()  [unwired: 1 in, 3 out]
      }
      event "模块启用配置": Value Change {
        n264 = event-data() -> ()  [unwired: 1 in, 6 out]
        n265 = call "模块启用配置框.vi"() -> ()  [unwired: 12 in]
      }
      event "24H周期设置", "运行模式", "多参数", "CODmn", "氨氮", "总氮", "CODCr", "质控启动日期", "空白核查时间", "跨度核查时间", "运行间隔", "周期设置", "流量阈值", "时间阈值", "总磷": Value Change {
        n266 = event-data() -> ()  [unwired: 1 in, 6 out]
        n267 = flat-sequence {
          frame #0 {
            n268 = local read "氨氮"() -> (w349:bool)
            n269 = local read "运行间隔"() -> (w340:i16)
            n270 = local read "流量阈值"() -> (w337:dbl)
            n271 = local read "周期设置"() -> (w339:enum16{"自由设定", "国标协议", "流量设定"})
            n272 = local read "时间阈值"() -> (w338:u16)
            n273 = local read "运行模式"() -> (w350:enum16{"维护模式", "常规模式", "应急模式", "质控模式"})
            n274 = local read "CODmn"() -> (w346:bool)
            n275 = local read "CODCr"() -> (w348:bool)
            n276 = local read "总氮"() -> (w336:bool)
            n277 = local read "总氮"() -> (w347:bool)
            n278 = local read "多参数"() -> (w345:bool)
            n279 = local read "空白核查时间"() -> (w342:u16)
            n280 = local read "质控启动日期"() -> (w343:string)
            n281 = local read "24H周期设置"() -> (w344:bool[])
            n282 = local read "跨度核查时间"() -> (w341:u16)
            n283 = global write "系统设置全局变量.vi" "氨氮自动启动设置"(w349) -> ()
            n284 = global write "系统设置全局变量.vi" "运行间隔"(w340) -> ()
            n285 = global write "系统设置全局变量.vi" "流量阈值"(w337) -> ()
            n286 = global write "系统设置全局变量.vi" "CODCr自动启动设置"(w348) -> ()
            n287 = global write "系统设置全局变量.vi" "周期设置"(w339) -> ()
            n288 = global write "系统设置全局变量.vi" "CODmn自动启动设置"(w346) -> ()
            n289 = global write "系统设置全局变量.vi" "时间阈值"(w338) -> ()
            n290 = global write "系统设置全局变量.vi" "多参数自动启动设置"(w345) -> ()
            n291 = global write "系统设置全局变量.vi" "运行模式"(w350) -> ()
            n292 = global write "系统设置全局变量.vi" "总磷自动启动设置"(w336) -> ()
            n293 = global write "系统设置全局变量.vi" "总氮自动启动设置"(w347) -> ()
            n294 = global write "系统设置全局变量.vi" "空白核查时间"(w342) -> ()
            n295 = global write "系统设置全局变量.vi" "质控启动日期"(w343) -> ()
            n296 = global write "系统设置全局变量.vi" "24H周期设置"(w344) -> ()
            n297 = global write "系统设置全局变量.vi" "跨度核查时间"(w341) -> ()
          }
          frame #1 {
            n298 = call <vilib>:"Application Directory.vi"() -> ("Application Directory"=w364:path)
            n299 = Build Path(base path=w364, name or relative path="data\\sys.ini" ("名称或相对路径")) -> (appended path=w362:path)
            n300 = call <vilib>:"Open Config Data.vi"("configuration file path"=w362) -> ("error out"=w358:errorcluster, "refnum"=w361:T1)  [unwired: 8 in, 1 out]
            n301 = vi-ref "系统设置全局变量.vi"() -> (w360:refnum<vi>)
            n302 = call <userlib>:"Write Panel to INI__ogtk.vi"("error in (no error)"=w358, "VI ref"=w360, "refnum"=w361) -> ("error out"=w357:errorcluster, "refnum out"=w359:T1)  [unwired: 7 in]
            n303 = call <vilib>:"Close Config Data.vi"("error in (no error)"=w357, "refnum"=w359) -> ("error out"=w352:errorcluster, "file path"=w351:path)  [unwired: 8 in]
            n304 = Open/Create/Replace File(file path (use dialog)=w351, error in=w352) -> (refnum out=w355:refnum<file>, error out=w356:errorcluster)  [unwired: 4 in, 1 out]
            n305 = Flush File(refnum=w355, error in=w356) -> (refnum out=w354:refnum<file>, error out=w353:errorcluster)
            n306 = Close File(refnum=w354, error in=w353) -> ()  [unwired: 2 out]
          }
        }
      }
      event "运行间隔": Mouse Down {
        n307 = event-data() -> ("CtlRef"=w368:refnum<vi>)  [unwired: 1 in, 7 out]
        n308 = property class="DigNum (严格)"(reference=w368) -> (reference out=w367:refnum<vi>, "Value"=w366:i16)  [unwired: 1 in, 1 out]
        n309 = call "数字键盘.vi"("OldNumber"=w366) -> ("NewNumber"=w365:sgl)
        n310 = property class="DigNum (严格)"(reference=w367, "Val(Sgnl)"=w365) -> ()  [unwired: 1 in, 2 out]
      }
      event "流量阈值": Mouse Down {
        n311 = event-data() -> ("CtlRef"=w372:refnum<vi>)  [unwired: 1 in, 7 out]
        n312 = property class="DigNum (严格)"(reference=w372) -> (reference out=w371:refnum<vi>, "Value"=w370:dbl)  [unwired: 1 in, 1 out]
        n313 = call "数字键盘.vi"("OldNumber"=w370) -> ("NewNumber"=w369:sgl)
        n314 = property class="DigNum (严格)"(reference=w371, "Val(Sgnl)"=w369) -> ()  [unwired: 1 in, 2 out]
      }
      event "时间阈值": Mouse Down {
        n315 = event-data() -> ("CtlRef"=w376:refnum<vi>)  [unwired: 1 in, 7 out]
        n316 = property class="DigNum (严格)"(reference=w376) -> (reference out=w375:refnum<vi>, "Value"=w374:u16)  [unwired: 1 in, 1 out]
        n317 = call "数字键盘.vi"("OldNumber"=w374) -> ("NewNumber"=w373:sgl)
        n318 = property class="DigNum (严格)"(reference=w375, "Val(Sgnl)"=w373) -> ()  [unwired: 1 in, 2 out]
      }
      event "开机启动": Value Change {
        n319 = event-data() -> ("NewVal"=w378:bool)  [unwired: 1 in, 5 out]
        n320 = call <vilib>:"Application Directory.vi"() -> ("Application Directory"=w377:path)
        n321 = case shown="真" w378 {
          tunnel: w377 -> [w380 w384]
          frame False {
            n322 = call "删除启动项.vi"("启动文件路径"=w380) -> ("删除标记"=w379:bool)  [unwired: 9 in, 1 out]
            n323 = case shown="真" w379 {
              frame False {
                n324 = local write "开机启动"(TRUE ("开机启动")) -> ()
                n325 = One Button Dialog(message="启动项删除失败" ("消息")) -> ()  [unwired: 1 in, 1 out]
              }
              frame True {
              }
            }
          }
          frame True {
            n326 = call "添加启动项.vi"("启动文件路径"=w384) -> ("添加成功标记"=w383:bool)  [unwired: 9 in, 1 out]
            n327 = case shown="真" w383 {
              frame False {
                n328 = local write "开机启动"(FALSE ("开机启动")) -> ()
                n329 = One Button Dialog(message="启动项添加失败" ("消息")) -> ()  [unwired: 1 in, 1 out]
              }
              frame True {
              }
            }
          }
        }
      }
      event "副屏显示设置": Value Change {
        n330 = event-data() -> ()  [unwired: 1 in, 6 out]
        n331 = call "副屏设置.vi"() -> ()  [unwired: 12 in]
      }
      event "首页显示设置": Value Change {
        n332 = event-data() -> ()  [unwired: 1 in, 6 out]
        n333 = call "首页显示设置.vi"() -> ()  [unwired: 12 in]
      }
      event "短信报警设置": Value Change {
        n334 = event-data() -> ()  [unwired: 1 in, 6 out]
        n335 = invoke class="VI" method="FP.Open"(reference=w389, "Activate"=TRUE ("激活？"), "State"=T5."Standard" ("状态")) -> ()  [unwired: 2 in, 5 out]
      }
      event "布尔": Value Change {
        n336 = event-data() -> ("OldVal"=w391:bool)  [unwired: 1 in, 5 out]
        n337 = case shown="假" w391 {
          tunnel: [w392 _] -> w390
          frame False {
            n338 = call "数字密码键盘.vi"() -> ("NewNumber"=w392:sgl)  [unwired: 1 in]
          }
          frame True {
          }
        }
        n339 = local write "输入密码"(w390) -> ()
      }
    }
  }
